vi "Lamis Hammouda Project 2 Code.vi"() -> ()   [LabVIEW 2020]
uses:
  <vilib>/MakerHub/LINX/LMH-LINX.lvlib
  <vilib>/Analysis/NI_AAL_SigProc.lvlib
  <vilib>/Analysis/3filter.llb/Filter Passband Type.ctl
  <vilib>/Analysis/NI_AALBase.lvlib
  <vilib>/MakerHub/LINX/Public/Peripherals/Analog/Analog Read 1 Chan.vi
  <vilib>/Analysis/3filter.llb/Butterworth Filter (DBL).vi
  <vilib>/MakerHub/LINX/Public/Peripherals/Digital/Digital Write N Chans.vi
panel:
  out "Filtered Subset \nPressure":dbl[](array[numeric])
  in  "Filter on?":bool=TRUE
  out "# valleys found":i32
  out "Valley Ampltidues":dbl[](array[numeric])
  out "Valley Locations":dbl[](array[numeric])
  in  "valley \nthreshold":dbl format="%0.2f"
  in  "valley width":i32=5 min=3
  in  "Write to File?":bool=TRUE
  in  "Filename":path=path "G:/My Drive/unc '24/3. Junior/Spring 2023/BMME 385/Project 2/Data/SubsetData.xlsx"
  out "MAP":dbl
  out "Peak Amplitudes":dbl[](array[numeric])
  out "Peak Locations":dbl[](array[numeric])
  out "# peaks found":i32
  in  "peak width":i32=5 min=3
  in  "peak \nthreshold":dbl format="%0.2f"
  out "Subset \nTimestamps":dbl[](array[numeric])
  out "Timestamps":dbl[](array[numeric])
  in  "send data":bool=TRUE
  in  "Digital Out Channels":u8[](array[numeric])=[10, 11, 12, 13]
  in  "digital out":bool[](array[boolean])=[FALSE, FALSE, FALSE, TRUE]
  in  "Stop Button":bool
  in  "AI Channel":u8
  in  "Serial Port":refnum<visa-resource-name>="COM10"
  out "array size actual":i32
  in  "Array Size (setting)":i32=20000
  out "Subset Pressure":dbl[](array[numeric])
  out "Pressure \nMonitor":cluster{dbl[], dbl[]}[](graph)
  out "BP Subset Monitor":cluster{dbl[], dbl[]}[](graph)
  in  "SUBSET DATA ENABLE":bool
  out "Pressure":dbl[](array[numeric]) format="%#_6f"
  # "PRESSURE MONITOR"
  # "SETTINGS"
  # "SUBSET DATA"
  # "PEAK DETECT"
  # "VALLEY DETECT"
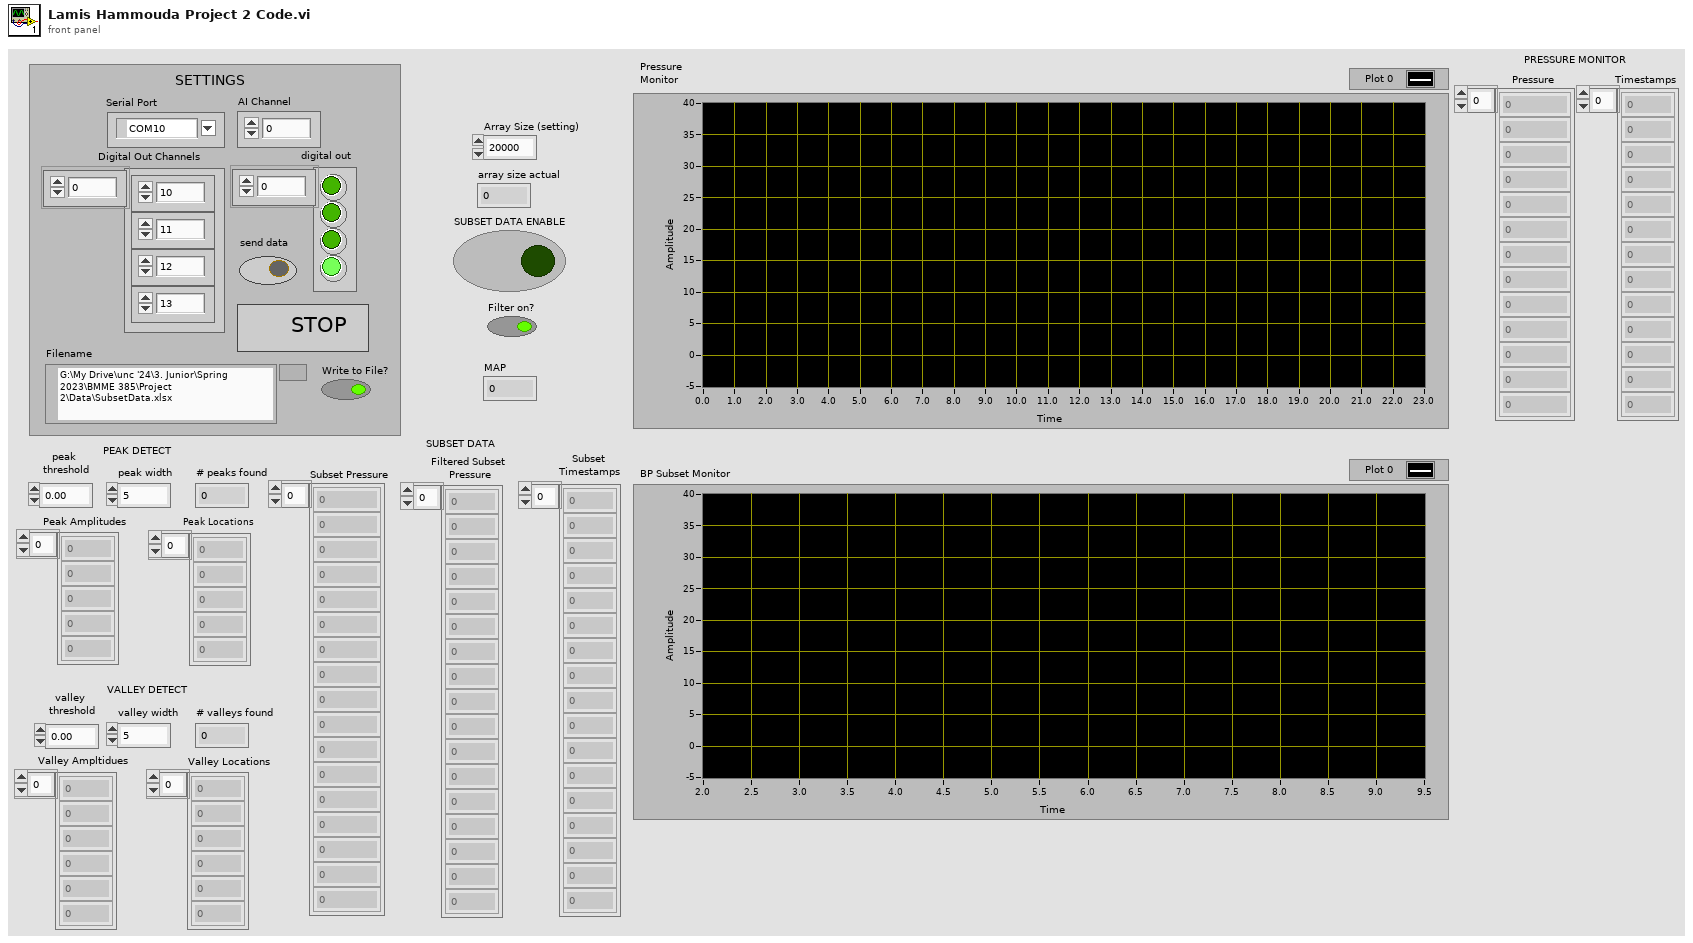
[diagram p1: front panel]
types:
  T1 = typedef "NI_AALBase.lvlib/Filter Passband Type.ctl" = enum32{"Lowpass", "Highpass", "Bandpass", "Bandstop"}
  T2 = typedef "LMH-LINX.lvlib/LINX Ref.ctl" = cluster{"IO":T3, "Interface":T4, "LINX Device Config":T5}
  T3 = typedef "LMH-LINX.lvlib/Platform.ctl" = enum16{"Remote", "Local"}
  T4 = typedef "LMH-LINX.lvlib/Interface.ctl" = enum16{"Serial", "TCP"}
  T5 = typedef "LMH-LINX.lvlib/Device.lvlib/LINX Device Config.ctl" = cluster{"Interface":T4, "COM Port":refnum<visa-resource-name>, "TCP Configuration":T6, "Device Family":u8, "Device ID":u8, "Device Name":string, "TCP Ref":refnum<k5>, "Channels":T7}
  T6 = typedef "LMH-LINX.lvlib/Device.lvlib/TCP Config.ctl" = cluster{"IP Address":string, "Port":u16}
  T7 = typedef "LMH-LINX.lvlib/Channels.ctl" = cluster{"DI":u8[], "DO":u8[], "AI":u8[], "AO":u8[], "PWM":u8[], "QE":u8[], "UART":u8[], "I2C 2":u8[], "SPI":u8[], "CAN":u8[], "Servo":u8[], "AI Ref (V)":dbl, "AI Resolution (Bits)":u8, "AO Ref (V)":dbl, "AO Resolution (Bits)":u8}
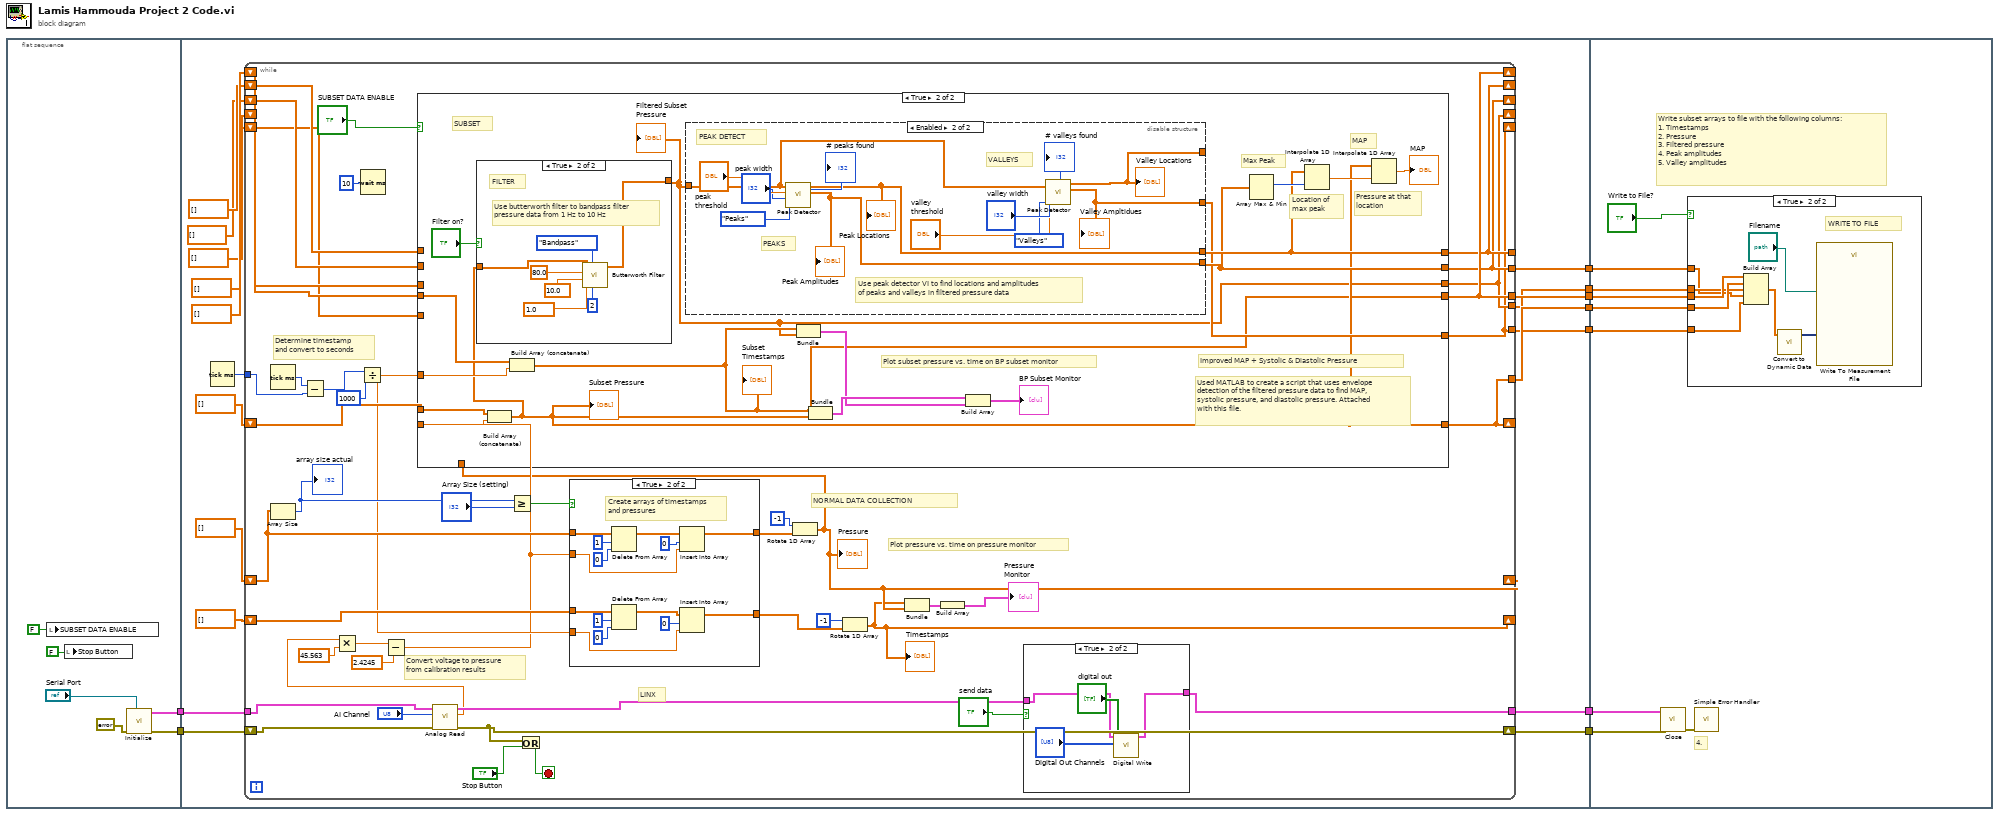
[diagram p0: block diagram]
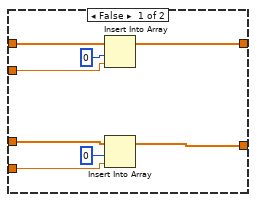
[diagram p3: hidden frame]
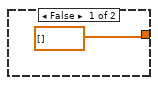
[diagram p5: hidden frame]
diagram:
  n1 = flat-sequence {
    tunnel: [w13] -> w9
    tunnel: [w12] -> w8
    tunnel: w9 -> [w28]
    tunnel: w8 -> [w27]
    tunnel: [w26] -> w7
    tunnel: [w25] -> w6
    tunnel: [w20] -> w5
    tunnel: [w19] -> w4
    tunnel: [w18] -> w3
    tunnel: [w17] -> w2
    tunnel: [w16] -> w1
    tunnel: w7 -> [w158]
    tunnel: w6 -> [w157]
    tunnel: w5 -> [w155]
    tunnel: w4 -> [w154]
    tunnel: w3 -> [w153]
    tunnel: w2 -> [w152]
    tunnel: w1 -> [w151]
    frame #0 {
      n2 = local write "SUBSET DATA ENABLE"(FALSE) -> ()
      n3 = local write "Stop Button"(FALSE) -> ()
      n4 = call <vilib>:"Initialize.vi"("Serial Port"="Serial Port", "Error In"=errorcluster {"status"=FALSE, "code"=0, "source"=""}) -> ("Error Out"=w12:errorcluster, "LINX Resource"=w13:T2)  [unwired: 7 in, 1 out]
    }
    frame #1 {
      n5 = Tick Count (ms)() -> (millisecond timer value=w33:u32)
      n6 = while {
        shift-right: [w37] -> _
        shift-left: dbl[] [] -> [w68]
        tunnel: w33 -> [w34]
        shift-right: [w35] -> _
        shift-left: dbl[] [] -> [w67]
        shift-right: [w46] -> _
        shift-left: dbl[] [] -> [w73]
        shift-right: [w36] -> _
        shift-left: dbl[] [] -> [w72]
        tunnel: w28 -> [w60]
        shift-right: [w57] -> w26
        shift-left: w27 -> [w61]
        tunnel: [w54] -> w25
        tunnel: [w46] -> w20
        tunnel: [w36] -> w19
        tunnel: [w40] -> w18
        tunnel: [w43] -> _
        tunnel: [w41] -> w17
        tunnel: [w38] -> w16
        shift-right: [w43] -> _
        shift-left: dbl[] [] -> [w45]
        shift-right: [w41] -> _
        shift-left: dbl[] [] -> [w42]
        shift-right: [w40] -> _
        shift-left: dbl[] [] -> [w44]
        shift-right: [w38] -> _
        shift-left: dbl[] [] -> [w39]
        stop <- w58 stop-if-true
        # "Determine timestamp \nand convert to seconds"
        # "Plot pressure vs. time on pressure monitor"
        # "Convert voltage to pressure \nfrom calibration results"
        # "LINX"
        # "NORMAL DATA COLLECTION"
        n7 = Tick Count (ms)() -> (millisecond timer value=w77:u32)
        n8 = Array Size(array=w68) -> (size(s)=w70:i32)
        "array size actual" <- w70
        n9 = Subtract(x=w77, y=w34) -> (x-y=w76:u32)
        n10 = Divide(x=w76, y=u32 1000) -> (x/y=w63:dbl)
        n11 = Wait (ms)(milliseconds to wait=u32 10) -> ()  [unwired: 1 out]
        n12 = call-poly <vilib>:"Analog Read.vi"("Error In"=w61, "Analog Channel"="AI Channel", "LINX Resource"=w60) -> ("Error Out"=w57:errorcluster, "Voltage"=w50:dbl, "LINX Resource"=w55:T2)  [unwired: 5 in, 1 out]
        n13 = Multiply(x=w50, y=45.563) -> (x*y=w53:dbl)
        n14 = Subtract(x=w53, y=2.4245) -> (x-y=w49:dbl)
        n15 = Greater Or Equal?(x=w70, y="Array Size (setting)") -> (x >= y?=w69:bool)
        n16 = Or(x=w57, y="Stop Button") -> (x .or. y?=w58:bool)
        n17 = case shown="True" w69 {
          tunnel: w49 -> [w92 w103]
          tunnel: w68 -> [w91 w106]
          tunnel: [w90 w100] -> w66
          tunnel: w67 -> [w87 w93]
          tunnel: [w86 w95] -> w65
          tunnel: w63 -> [w85 w94]
          frame False {
            n18 = Insert Into Array(array=w91, index=0, new element=w92) -> (w90:dbl[])
            n19 = Insert Into Array(array=w87, index=0, new element=w85) -> (w86:dbl[])
          }
          frame True {
            # "Create arrays of timestamps\nand pressures"
            n20 = Delete From Array(array=w106, length=1, index=0) -> (array with subset deleted=w101:dbl[])  [unwired: 1 out]
            n21 = Delete From Array(array=w93, length=1, index=0) -> (array with subset deleted=w96:dbl[])  [unwired: 1 out]
            n22 = Insert Into Array(array=w101, index=0, new element=w103) -> (w100:dbl[])
            n23 = Insert Into Array(array=w96, index=0, new element=w94) -> (w95:dbl[])
          }
        }
        n24 = Rotate 1D Array(1:w66, 2:-1 ("n")) -> (0:w37:dbl[])
        "Pressure" <- w37
        n25 = case shown="True" "SUBSET DATA ENABLE" {
          tunnel: w73 -> [w112 w129]
          tunnel: [w112 w114] -> w46
          tunnel: w63 -> [_ w128]
          tunnel: w72 -> [w111 w127]
          tunnel: w49 -> [_ w126]
          tunnel: [w111 w115] -> w36
          tunnel: [w108 w113] -> w40
          tunnel: [w110 w119] -> w43
          tunnel: [w109 w118] -> w41
          tunnel: [w107 w117] -> w38
          tunnel: w45 -> [w110 _]
          tunnel: w42 -> [w109 _]
          tunnel: w44 -> [w108 _]
          tunnel: w39 -> [w107 _]
          tunnel: w37 -> [_ _]
          frame False {
          }
          frame True {
            # "Plot subset pressure vs. time on BP subset monitor"
            # "Pressure at that\nlocation"
            # "Location of \nmax peak"
            # "Max Peak"
            # "Used MATLAB to create a script that uses envelope\ndetection of the filtered pressure data to find MAP,\nsystolic pressure, and diastolic pressure. Attached\nwith this file."
            # "Improved MAP + Systolic & Diastolic Pressure"
            # "MAP"
            # "SUBSET"
            n26 = Build Array (concatenate)(w127, w126) -> (w115:dbl[])
            "Subset Pressure" <- w115
            n27 = case shown="True" "Filter on?" {
              tunnel: w115 -> [_ w137]
              tunnel: [dbl[] [] ("Filtered X") w131] -> w113
              frame False {
              }
              frame True {
                # "Use butterworth filter to bandpass filter\npressure data from 1 Hz to 10 Hz"
                # "FILTER"
                n28 = call-poly <vilib>:"Butterworth Filter.vi"("order"=2, "filter type"=Filter_Passband_Type."Bandpass", "low cutoff freq: fl"=1.0, "high cutoff freq: fh"=10.0, "sampling freq: fs"=80.0, "X"=w137) -> ("Filtered X"=w131:dbl[])  [unwired: 2 in, 1 out]
              }
            }
            "Filtered Subset \nPressure" <- w113
            n29 = Build Array (concatenate)(w129, w128) -> (w114:dbl[])
            "Subset \nTimestamps" <- w114
            n30 = disable-structure shown="Enabled" {
              disable-tunnel: w113 -> [_ w141]
              disable-tunnel: [_ w146] -> w119
              disable-tunnel: [_ w145] -> w118
              disable-tunnel: [_ w140] -> w117
              disable-tunnel: [_ w138] -> _
              frame Disabled {
              }
              frame Enabled {
                # "Use peak detector VI to find locations and amplitudes\nof peaks and valleys in filtered pressure data"
                # "VALLEYS"
                # "PEAKS"
                # "PEAK DETECT"
                n31 = call <vilib>:"Peak Detector.vi"("peaks/valleys"=enum32{"Peaks", "Valleys"}."Peaks", "width"="peak width", "threshold"="peak \nthreshold", "X"=w141) -> ("Amplitudes"=w145:dbl[], "Locations"=w146:dbl[], "# found"=→"# peaks found":i32)  [unwired: 3 in, 2 out]
                "Peak Locations" <- w146
                "Peak Amplitudes" <- w145
                n32 = call <vilib>:"Peak Detector.vi"("peaks/valleys"=enum32{"Peaks", "Valleys"}."Valleys", "width"="valley width", "threshold"="valley \nthreshold", "X"=w141) -> ("Amplitudes"=w140:dbl[], "Locations"=w138:dbl[], "# found"=→"# valleys found":i32)  [unwired: 3 in, 2 out]
                "Valley Locations" <- w138
                "Valley Ampltidues" <- w140
              }
            }
            n33 = Bundle(w114, "Filtered X"=w113) -> (w123:cluster{dbl[], "Filtered X":dbl[]})  [unwired: 1 in]
            n34 = Bundle(w114, w115) -> (w125:cluster{dbl[], dbl[]})  [unwired: 1 in]
            n35 = Build Array(w125, w123) -> (→"BP Subset Monitor":cluster{dbl[], "Filtered X":dbl[]}[])
            n36 = Array Max & Min(array=w118) -> (max index (indices)=w120:i32)  [unwired: 3 out]
            n37 = Interpolate 1D Array(1:w120, 2:w119) -> (0:w122:dbl)
            n38 = Interpolate 1D Array(1:w122, 2:w115) -> (0:→"MAP":dbl)
          }
        }
        n39 = Rotate 1D Array(1:w65, 2:-1 ("n")) -> (0:w35:dbl[])
        "Timestamps" <- w35
        n40 = Bundle(w35, w37) -> (w47:cluster{dbl[], dbl[]})  [unwired: 1 in]
        n41 = Build Array(w47) -> (→"Pressure \nMonitor":cluster{dbl[], dbl[]}[])
        n42 = case shown="True" "send data" {
          tunnel: [w80 w84] -> w54
          tunnel: w55 -> [w80 w81]
          frame False {
          }
          frame True {
            n43 = call-poly <vilib>:"Digital Write.vi"("Values"="digital out", "DO Channels"="Digital Out Channels", "LINX Resource"=w81) -> ("LINX Resource"=w84:T2)  [unwired: 7 in, 1 out]
          }
        }
      }
    }
    frame #2 {
      # "Write subset arrays to file with the following columns:\n1. Timestamps\n2. Pressure\n3. Filtered pressure\n4. Peak amplitudes\n5. Valley amplitudes"
      # "4."
      n44 = call <vilib>:"Close.vi"("Error In"=w158, "LINX Resource"=w157) -> ("Error Out"=w159:errorcluster)  [unwired: 9 in]
      n45 = case shown="True" "Write to File?" {
        tunnel: w155 -> [_ w164]
        tunnel: w154 -> [_ w163]
        tunnel: w153 -> [_ w162]
        tunnel: w152 -> [_ w161]
        tunnel: w151 -> [_ w160]
        frame False {
        }
        frame True {
          # "WRITE TO FILE"
          n46 = Build Array(w164, w163, w162, w161, w160) -> (w167:dbl[][])
          n47 = call "Convert to Dynamic Data"("2D Array"=w167) -> ("Dynamic Data Type"=w165:dynamicdata)  [unwired: 3 in]
          n48 = call "Write To Measurement File"("Signals"=w165, "Filename"="Filename") -> ()  [unwired: 15 in, 3 out]
        }
      }
      n49 = call <vilib>:"Simple Error Handler.vi"("error in (no error)"=w159) -> ()  [unwired: 4 in, 5 out]
    }
  }
